vi "Clear Multiple Errors.vi"(8 "Error In":errorcluster, 11 "Errors to Clear":i32[](array[numeric])=[0]) -> (0 "Error Out":errorcluster, 3 "Specific Errors Cleared?":bool)   [LabVIEW 2013, in "TS.lvlib"]
doc: "This VI behaves much like the built-in\nClear Errors.vi, but allows an array of\ninput errors to clear. If any of them are\ncleared, the Specific Errors Cleared? is set to TRUE.\nThe Errors to Clear array has a default of a single\nvalue set to 0 to mimic the behavior of the NI version."
uses:
  TS.lvlib
panel:
  # "This VI behaves much like the built-in\nClear Errors.vi, but allows an array of\ninput errors to clear. If any of them are\ncleared, the Specific Errors Cleared? is set to TRUE.\nThe Errors to Clear array has a default of a single\nvalue set to 0 to mimic the behavior of the NI version."
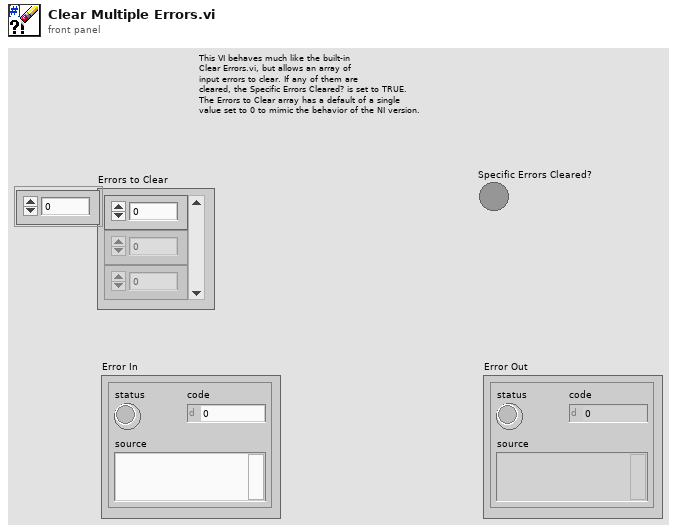
[diagram p1: front panel]
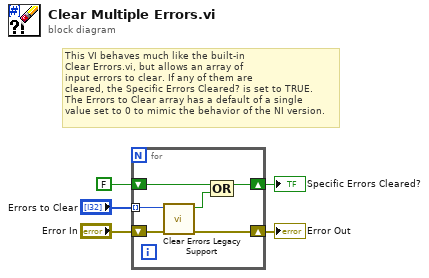
[diagram p0: block diagram]
diagram:
  # "This VI behaves much like the built-in\nClear Errors.vi, but allows an array of\ninput errors to clear. If any of them are\ncleared, the Specific Errors Cleared? is set to TRUE.\nThe Errors to Clear array has a default of a single\nvalue set to 0 to mimic the behavior of the NI version."
  n1 = for {
    tunnel: "Errors to Clear" -> [w11] mode=indexing
    shift-right: [w8] -> w3
    shift-left: FALSE -> [w10]
    shift-right: [w6] -> w1
    shift-left: "Error In" -> [w7]
    n2 = call "Clear Errors Legacy Support.vi"("error in (no error)"=w7, "specific error code to clear (0: all)"=w11) -> ("error out"=w6:errorcluster, "specific error cleared?"=w9:bool)  [unwired: 4 in]
    n3 = Compound Arithmetic op=OR(w10, w9) -> (w8:bool)
  }
  "Error Out" <- w1
  "Specific Errors Cleared?" <- w3
